vi "数组拼回字符串.vi"(5 "数组":string[](array[string])) -> (2 "字符串":string)   [LabVIEW 2016, in "TCP接收文件.lvlib"]
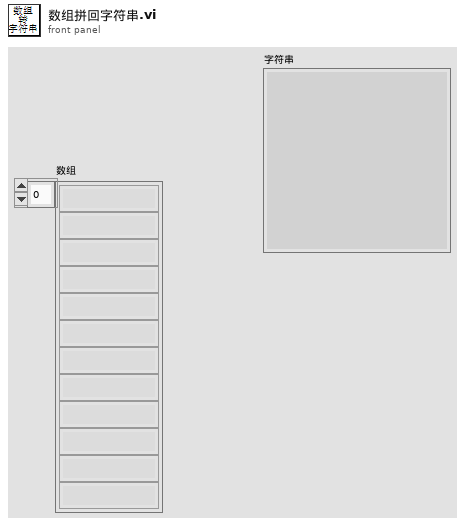
[diagram p1: front panel]
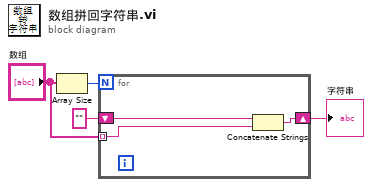
[diagram p0: block diagram]
diagram:
  n1 = Array Size(array="数组") -> (size(s)=w4:i32)
  n2 = for {
    N: w4 -> [_]
    shift-right: [w7] -> w3
    shift-left: "" -> [w6]
    tunnel: "数组" -> [w5] mode=indexing
    n3 = Concatenate Strings(w6, w5) -> (w7:string)
  }
  "字符串" <- w3
